vi "Rinocloud_real-time_monitoring.vi"() -> ()   [LabVIEW 2013, in "Rinocloud Library.lvlib"]
uses:
  Rinocloud Library.lvlib
  Rinocloud_global_variable.vi
  Rinocloud API endpoint VIs/API_endpoint_subVIs/Rinocloud_get_metadata_field_value_subVIs/get_numeric_value.vi
  Rinocloud API endpoint VIs/API_endpoint_subVIs/Rinocloud_get_metadata_field_value_subVIs/get_string_value.vi
panel:
  out "Local status:":string="OFF"
  in  "Toggle":bool
  out "Sending...":bool
  out "System Waveform Graph":dbl[](graph)
  out "Data chunk":string
  in  "Record name":string
  in  "create empty":bool
  in  "Request period (s)":dbl=1.0 format="%#.2f"
  out "Remote status:":string="OFF"
  in  "stop":bool
  out "Parent folder:":string
  # "Request period and measurement status\ncan be set remotely by\n{\"period\":<value in s>, \"status\":\"on<or off>\"}\n\nLocal changes of period or/and status are \nupdated immediatelly on Rinocloud."
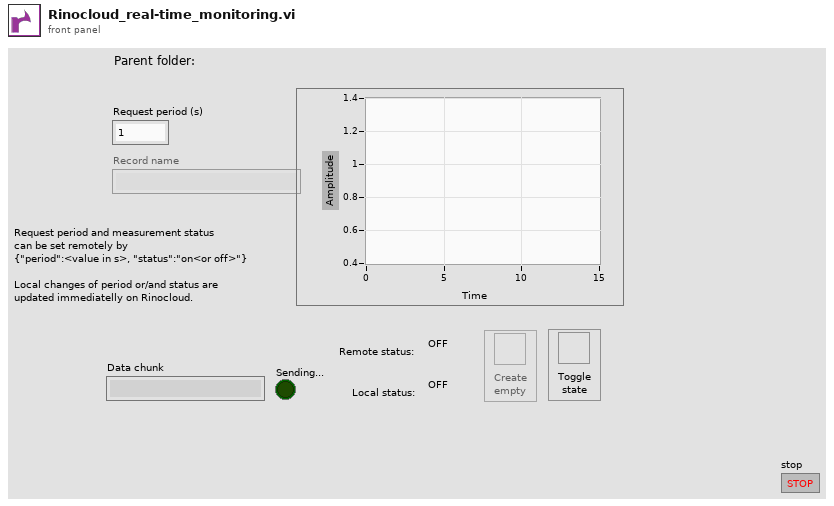
[diagram p1: front panel]
types:
  T1 = cluster{"Record ID":string, "Status":string, "Record name":string, "Parent ID":string, "Request period (s)":dbl, "Sending...":bool, "Parent folder":string, "HTTP resp body":string, "Data chunk":string, "error out":errorcluster, "error in (no error)":errorcluster, "x":dbl, "y array":dbl[], "y":dbl}
  T2 = enum16{"initialize", "create empty", "append", "wait for event", "start append", "generate data"}
  T3 = enum8{"Enabled", "Disabled", "Disabled and Grayed Out"}
  T4 = enum16{"initialize", "create empty", "append", "wait for event"}
  T5 = cluster{"Attribute":string, "Value":string, "Data type":enum16{"Numeric", "String", "1D array of strings", "1D array of doubles", "Data JSON string", "<null>"}}
  T6 = enum16{"Numeric", "String", "1D array of strings", "1D array of doubles", "Data JSON string", "<null>"}
  T7 = cluster{"Attribute":string, "Value":string, "Data type":enum16{"Numeric", "String", "1D array of strings", "1D array of doubles", "Data JSON string", "<null>"}}[]
  T8 = cluster{"headers":string, "body":string, "ID":string, "Saved":bool}
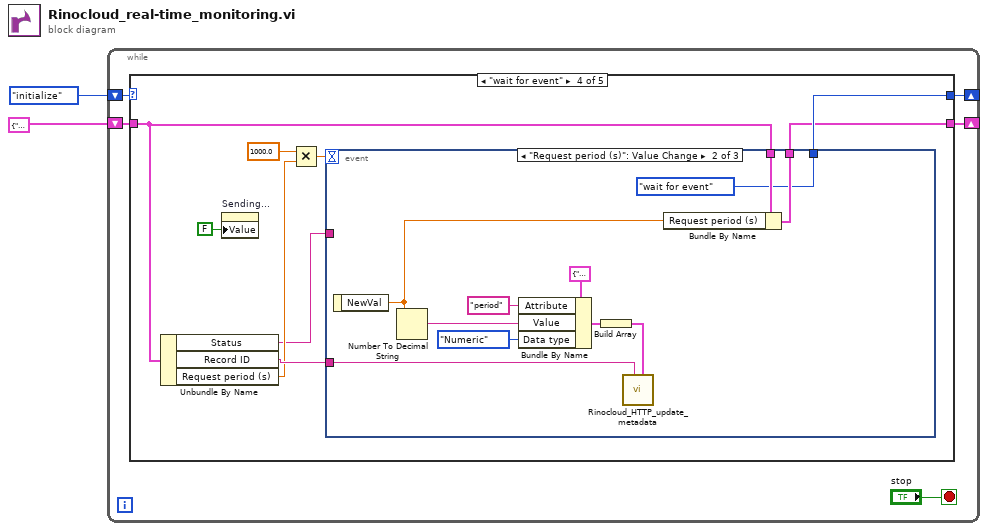
[diagram p0: block diagram]
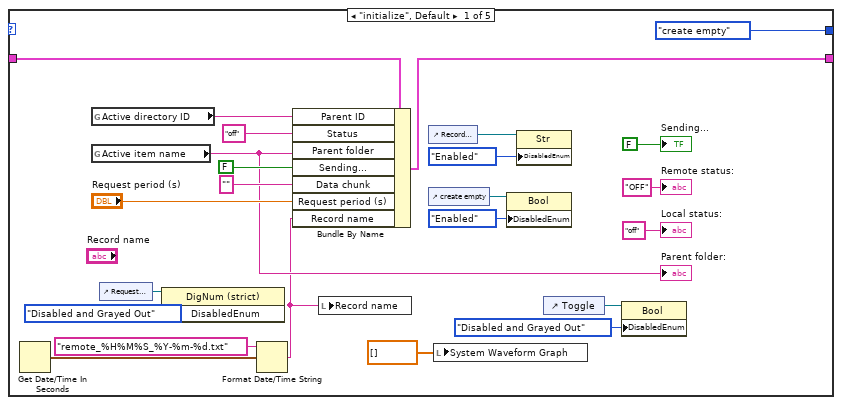
[diagram p2: hidden frame]
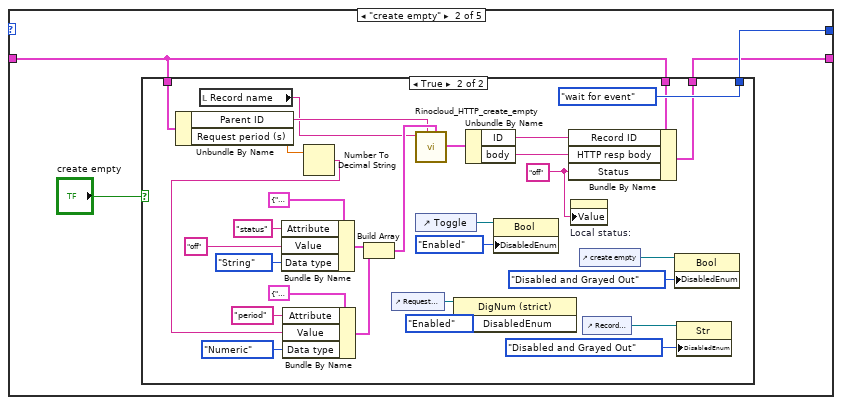
[diagram p3: hidden frame]
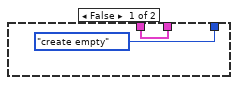
[diagram p4: hidden frame]
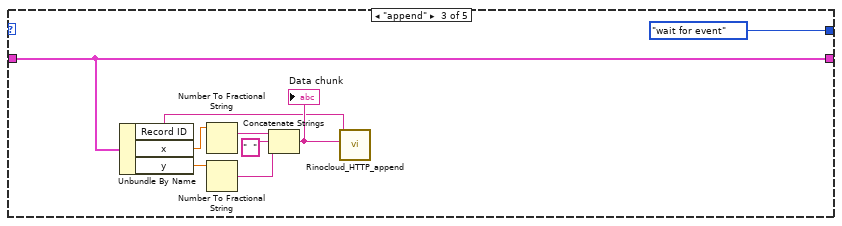
[diagram p5: hidden frame]
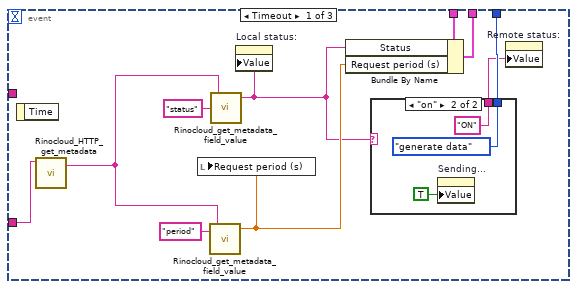
[diagram p6: hidden frame]
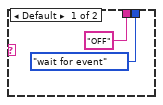
[diagram p7: hidden frame]
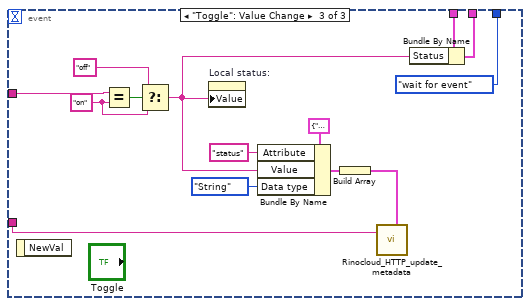
[diagram p8: hidden frame]
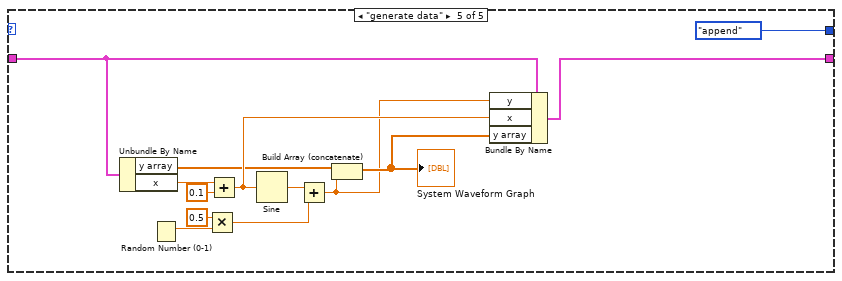
[diagram p9: hidden frame]
diagram:
  n1 = while {
    shift-right: [w3] -> _
    shift-left: T2."initialize" -> [w4]
    shift-right: [w5] -> _
    shift-left: T1 {"Record ID"="", "Status"="", "Record name"="", "Parent ID"="", "Request period (s)"=1.0, "Sending..."=FALSE, "Parent folder"="", "HTTP resp body"="", "Data chunk"="", "error out"={"status"=FALSE, "code"=0, "source"=""}, "error in (no error)"={"status"=FALSE, "code"=0, "source"=""}, "x"=0.0, "y array"=[], "y"=0.0} ("Cluster") -> [w6]
    stop <- "stop" stop-if-true
    n2 = case shown="\"wait for event\"" w4 {
      tunnel: [w30 w32 w68 w79 w128] -> w5
      tunnel: w6 -> [w31 w33 w68 w80 w129]
      tunnel: [T4."create empty" w35 T2."wait for event" w81 T2."append"] -> w3
      frame "initialize", Default {
        n3 = Get Date/Time In Seconds() -> (seconds since 1Jan1904=w14:timestamp)
        n4 = global read "Rinocloud_global_variable.vi" "Active directory ID"() -> (w28:string)
        n5 = global read "Rinocloud_global_variable.vi" "Active item name"() -> (w24:string)
        "Parent folder:" <- w24
        n6 = control-ref of="Request period (s)"() -> (w8:refnum<vi>)
        n7 = property class="DigNum (strict)"(reference=w8, "DisabledEnum"=T3."Disabled and Grayed Out" ("Disabled")) -> ()  [unwired: 1 in, 2 out]
        n8 = Format Date/Time String(time format string (%c)="remote_%H%M%S_%Y-%m-%d.txt", seconds (now)=w14) -> (date/time string=w12:string)  [unwired: 1 in]
        n9 = Bundle By Name(cluster=w31, "Parent ID"=w28, "Status"="off", "Parent folder"=w24, "Sending..."=FALSE, "Data chunk"="", "Request period (s)"="Request period (s)", "Record name"=w12) -> (w30:T1)
        n10 = local write "Record name"(w12) -> ()
        n11 = control-ref of="Record name"() -> (w15:refnum<vi>)
        n12 = control-ref of="create empty"() -> (w22:refnum<vi>)
        n13 = local write "System Waveform Graph"(dbl[] [] ("y array")) -> ()
        n14 = property class="Bool"(reference=w22, "DisabledEnum"=T3."Enabled" ("Disabled")) -> ()  [unwired: 1 in, 2 out]
        n15 = property class="Str"(reference=w15, "DisabledEnum"=T3."Enabled" ("Disabled")) -> ()  [unwired: 1 in, 2 out]
        n16 = control-ref of="Toggle"() -> (w10:refnum<vi>)
        n17 = property class="Bool"(reference=w10, "DisabledEnum"=T3."Disabled and Grayed Out" ("Disabled")) -> ()  [unwired: 1 in, 2 out]
        "Remote status:" <- "OFF" ("Status:")
        "Sending..." <- FALSE ("Sending...")
        "Local status:" <- "off" ("Status:")
      }
      frame "create empty" {
        n18 = case shown="True" "create empty" {
          tunnel: [T4."create empty" T4."wait for event"] -> w35
          tunnel: w33 -> [_ w59]
          tunnel: w33 -> [w36 w57]
          tunnel: [w36 w56] -> w32
          frame False {
          }
          frame True {
            w45 = "off" ("Status:")
            n19 = Unbundle By Name(w59) -> ("Parent ID"=w58:string, "Request period (s)"=w48:dbl)
            n20 = local read "Record name"() -> (w42:string)
            n21 = Bundle By Name(cluster=T5 {"Attribute"="", "Value"="", "Data type"=enum."<null>"} ("extra information field 4"), "Attribute"="status", "Value"="off", "Data type"=T6."String") -> (w63:T5)
            n22 = Number To Decimal String(number=w48) -> (decimal integer string=w47:string)  [unwired: 1 in]
            n23 = Bundle By Name(cluster=T5 {"Attribute"="", "Value"="", "Data type"=enum."<null>"} ("extra information field 4"), "Attribute"="period", "Value"=w47, "Data type"=T6."Numeric") -> (w46:T5)
            n24 = Build Array(w63, w46) -> (w62:T7)
            n25 = control-ref of="Request period (s)"() -> (w38:refnum<vi>)
            n26 = call "Rinocloud_HTTP_create_empty.vi"("Extra metadata array"=w62, "Parent ID"=w58, "Name"=w42) -> ("Status"=w61:T8)  [unwired: 5 in, 1 out]
            n27 = control-ref of="Toggle"() -> (w40:refnum<vi>)
            n28 = property class="DigNum (strict)"(reference=w38, "DisabledEnum"=T3."Enabled" ("Disabled")) -> ()  [unwired: 1 in, 2 out]
            n29 = Unbundle By Name(w61) -> ("ID"=w55:string, "body"=w54:string)
            n30 = property class="Bool"(reference=w40, "DisabledEnum"=T3."Enabled" ("Disabled")) -> ()  [unwired: 1 in, 2 out]
            n31 = Bundle By Name(cluster=w57, "Record ID"=w55, "HTTP resp body"=w54, "Status"=w45) -> (w56:T1)
            n32 = property on="Local status:" class="Str"("Value"=w45) -> ()  [unwired: 2 in, 2 out]
            n33 = control-ref of="create empty"() -> (w53:refnum<vi>)
            n34 = control-ref of="Record name"() -> (w44:refnum<vi>)
            n35 = property class="Bool"(reference=w53, "DisabledEnum"=T3."Disabled and Grayed Out" ("Disabled")) -> ()  [unwired: 1 in, 2 out]
            n36 = property class="Str"(reference=w44, "DisabledEnum"=T3."Disabled and Grayed Out" ("Disabled")) -> ()  [unwired: 1 in, 2 out]
          }
        }
      }
      frame "append" {
        n37 = Unbundle By Name(w68) -> ("Record ID"=w71:string, "x"=w72:dbl, "y"=w70:dbl)
        n38 = Number To Fractional String(number=w72) -> (F-format string=w74:string)  [unwired: 3 in]
        n39 = Number To Fractional String(number=w70) -> (F-format string=w76:string)  [unwired: 3 in]
        n40 = Concatenate Strings(w74, "  " ("string"), w76) -> (w73:string)
        "Data chunk" <- w73
        n41 = call "Rinocloud_HTTP_append.vi"("chunk"=w73, "ID"=w71) -> ()  [unwired: 4 in, 3 out]
      }
      frame "wait for event" {
        n42 = Unbundle By Name(w80) -> ("Status"=w78:string, "Record ID"=w85:string, "Request period (s)"=w83:dbl)
        n43 = property on="Sending..." class="Bool (strict)"("Value"=FALSE ("Sending...")) -> ()  [unwired: 2 in, 2 out]
        n44 = Multiply(x=1000.0, y=w83) -> (x*y=w84:dbl)
        n45 = event shown="[1] \"Request period (s)\": Value Change" {
          selector: _ -> [_ _ _]
          dyn-events: _ -> [_ _ _]
          timeout: w84 -> [_ _ _]
          tunnel: w85 -> [w94 w101 w117]
          tunnel: [w93 T2."wait for event" T2."wait for event"] -> w81
          tunnel: w80 -> [w91 w111 w115]
          tunnel: [w90 w110 w114] -> w79
          tunnel: w78 -> [_ _ w125]
          event Timeout {
            n46 = event-data() -> ()  [unwired: 1 in, 1 out]
            n47 = call "Rinocloud_HTTP_get_metadata.vi"("id"=w94) -> ("metadata (JSON)"=w86:string)  [unwired: 4 in, 6 out]
            n48 = call-poly "Rinocloud_get_metadata_field_value.vi"("field name"="period", "metadata JSON string"=w86) -> ("field value"=w88:dbl)  [unwired: 2 in, 1 out]
            n49 = local write "Request period (s)"(w88) -> ()
            n50 = call-poly "Rinocloud_get_metadata_field_value.vi"("field name"="status" ("Parameter Name"), "metadata JSON string"=w86) -> ("field value"=w87:string)  [unwired: 2 in, 1 out]
            n51 = property on="Local status:" class="Str"("Value"=w87) -> ()  [unwired: 2 in, 2 out]
            n52 = Bundle By Name(cluster=w91, "Status"=w87, "Request period (s)"=w88) -> (w90:T1)
            n53 = case shown="\"on\"" w87 {
              tunnel: [T2."wait for event" T2."generate data"] -> w93
              tunnel: ["OFF" ("Parameter Name") "ON" ("Parameter Name")] -> w92
              frame Default {
              }
              frame "on" {
                n54 = property on="Sending..." class="Bool (strict)"("Value"=TRUE ("Sending...")) -> ()  [unwired: 2 in, 2 out]
              }
            }
            n55 = property on="Remote status:" class="Str"("Value"=w92) -> ()  [unwired: 2 in, 2 out]
          }
          event "Request period (s)": Value Change {
            n56 = event-data() -> ("NewVal"=w104:dbl)  [unwired: 1 in]
            n57 = Number To Decimal String(number=w104) -> (decimal integer string=w105:string)  [unwired: 1 in]
            n58 = Bundle By Name(cluster=T5 {"Attribute"="", "Value"="", "Data type"=enum."<null>"} ("extra information field 4"), "Attribute"="period", "Value"=w105, "Data type"=T6."Numeric") -> (w103:T5)
            n59 = Build Array(w103) -> (w102:T7)
            n60 = call "Rinocloud_HTTP_update_metadata.vi"("Extra metadata array"=w102, "self ID"=w101) -> ()  [unwired: 8 in, 2 out]
            n61 = Bundle By Name(cluster=w111, "Request period (s)"=w104) -> (w110:T1)
          }
          event "Toggle": Value Change {
            w113 = "on" ("y")
            n62 = event-data() -> ()  [unwired: 1 in, 1 out]
            n63 = Equal?(x=w125, y=w113) -> (x = y?=w119:bool)
            n64 = Select(t="off" ("y"), s=w119, f=w113) -> (s? t:f=w112:string)
            n65 = property on="Local status:" class="Str"("Value"=w112) -> ()  [unwired: 2 in, 2 out]
            n66 = Bundle By Name(cluster=T5 {"Attribute"="", "Value"="", "Data type"=enum."<null>"} ("extra information field 4"), "Attribute"="status", "Value"=w112, "Data type"=T6."String") -> (w121:T5)
            n67 = Build Array(w121) -> (w120:T7)
            n68 = call "Rinocloud_HTTP_update_metadata.vi"("Extra metadata array"=w120, "self ID"=w117) -> ()  [unwired: 8 in, 2 out]
            n69 = Bundle By Name(cluster=w115, "Status"=w112) -> (w114:T1)
          }
        }
      }
      frame "generate data" {
        n70 = Unbundle By Name(w129) -> ("y array"=w131:dbl[], "x"=w130:dbl)
        n71 = Random Number (0-1)() -> (number: 0 to 1=w137:dbl)
        n72 = Multiply(x=0.5, y=w137) -> (x*y=w134:dbl)
        n73 = Add(x=w130, y=0.1) -> (x+y=w133:dbl)
        n74 = Sine(x=w133) -> (sin(x)=w135:dbl)
        n75 = Add(x=w135, y=w134) -> (x+y=w127:dbl)
        n76 = Build Array (concatenate)(w131, w127) -> (w132:dbl[])
        "System Waveform Graph" <- w132
        n77 = Bundle By Name(cluster=w129, "y"=w127, "x"=w133, "y array"=w132) -> (w128:T1)
      }
    }
  }
